vi "Vision Research Phantom Series PhFile PhStopWriteCineFileAsync.vi"(0 "CH [in]":u64, 5 "Error In (no error)":errorcluster) -> (19 "Error Out":errorcluster)   [LabVIEW 2013, in "VRI.lvlib"]
doc: "PhStopWriteCineFileAsync\nHRESULT PhStopWriteCineFileAsync(CINEHANDLE CH);\n\nParameters\nCH [in]\n Cine handle.\n\nReturn Value\nThe function returns ERR_Ok in case of success or an error code, otherwise. To get extended error information call PhGetErrorMessage.\n\nRemarks\nStops an asynchronous save operation for the specified cine.\n\nRequired Header\nPhFile.h"
uses:
  VRI.lvlib
  Phantom DLLs/PhFile.dll
panel:
  # "For instructions on the use of this VI, press Ctrl+H to display the help window and move the mouse over the icon, controls, and indicators"
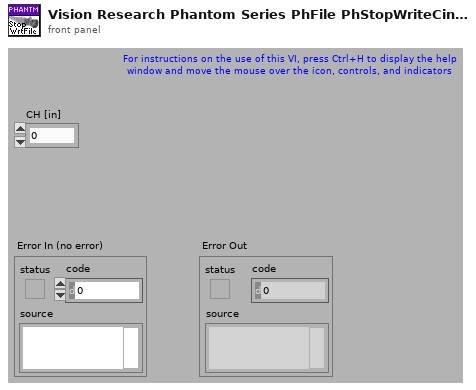
[diagram p1: front panel]
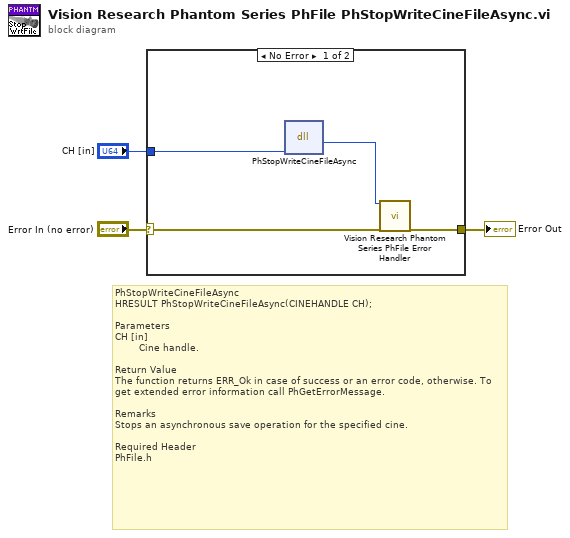
[diagram p0: block diagram]
diagram:
  # "PhStopWriteCineFileAsync\nHRESULT PhStopWriteCineFileAsync(CINEHANDLE CH);\n\nParameters\nCH [in]\n        Cine handle.\n\nReturn Value\nThe function returns ERR_Ok in case of success or an error code, otherwise. To get extended error information call PhGetErrorMessage.\n\nRemarks\nStops an asynchronous save operation for the specified cine.\n\nRequired Header\nPhFile.h"
  n1 = case shown="No Error" "Error In (no error)" {
    selector: "Error In (no error)" -> [w7 w8]
    tunnel: [w6 w8] -> w2
    tunnel: "CH [in]" -> [w5 _]
    frame No Error {
      n2 = dll-call lib="C:/Projects/SDK/32-bit/Vision Research Phantom Series Labview Driver/Phantom DLLs/PhFile.dll" fn="PhStopWriteCineFileAsync"("CH"=w5) -> ("HRESULT"=w4:i32)  [unwired: 4 in, 2 out]
      n3 = call "Vision Research Phantom Series PhFile Error Handler.vi"("Error Code (0)"=w4, "Error In (no error)"=w7) -> ("Error Out"=w6:errorcluster)  [unwired: 17 out]
    }
    frame Error {
    }
  }
  "Error Out" <- w2
